vi "mergeFractionalSeconds[us].vi"(9 "Fractional Second":dbl format="%#.6f", 10 "(Integer) Time (s)":i64, 11 "Epoch in":refnum<class "Epoch.lvclass">) -> (2 "(Integer) Time (us)":i64, 3 "Epoch out":refnum<class "Epoch.lvclass">)   [LabVIEW 2013, in "Epoch.lvclass"]
uses:
  Epoch.lvclass
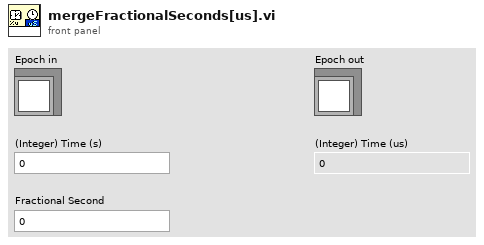
[diagram p1: front panel]
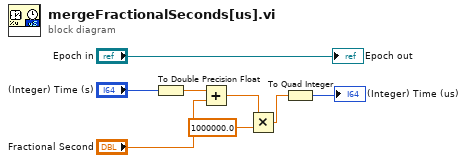
[diagram p0: block diagram]
diagram:
  n1 = To Double Precision Float(number="(Integer) Time (s)") -> (double precision float=w5:dbl)
  n2 = Add(x=w5, y="Fractional Second") -> (x+y=w3:dbl)
  n3 = Multiply(x=w3, y=1000000.0) -> (x*y=w2:dbl)
  n4 = To Quad Integer(1:w2) -> (0:→"(Integer) Time (us)":i64)
  "Epoch out" <- "Epoch in"
